vi "controlLaw_deltaU_distEst.vi"(7 "Control Params":T1={"umax"=3.0, "y_ref(k)"=0.0, "Ki"=0.0, "y(k) (from plant)"=0.0, "ND"=0, "NS"=0, "u_Kx_ref(k)"=0.0, "du_max"=3.0, "NS_obs"=0, "NS_control"=0} {"du_max" format="%#_13g"; "u_Kx_ref(k)" format="%#_13g"; "Ki" format="%#_13g"; "y_ref(k)" format="%#_13g"; "umax" format="%#_13g"}, 8 "x^(k)":sgl[](array[numeric])=[0.0, 0.0, 0.0, 0.0, 0.0, 0.0, 0.0, 0.0, 0.0, 0.0, 0.0, 0.0, 0.0, 0.0, 0.0, 0.0, 0.0, 0.0, 0.0, 0.0, 0.0, 0.0, 0.0, 0.0, 0.0]) -> (0 "x^(k+1) = Ax + Bu + Lye":sgl[](array[numeric]), 3 "u(k) (saturated)":sgl)   [LabVIEW 2017]
uses:
  controls/controlParams_tracktraj.ctl
panel:
  out "has_saturated":bool
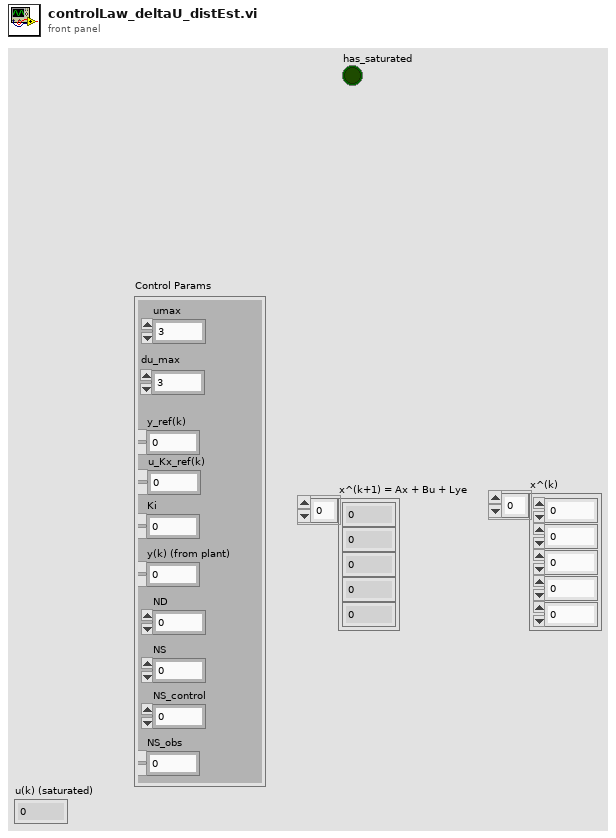
[diagram p1: front panel]
types:
  T1 = typedef "controlParams_tracktraj.ctl" = cluster{"umax":sgl, "y_ref(k)":sgl, "Ki":sgl, "y(k) (from plant)":sgl, "ND":i16, "NS":i16, "u_Kx_ref(k)":sgl, "du_max":sgl, "NS_obs":i16, "NS_control":i16}
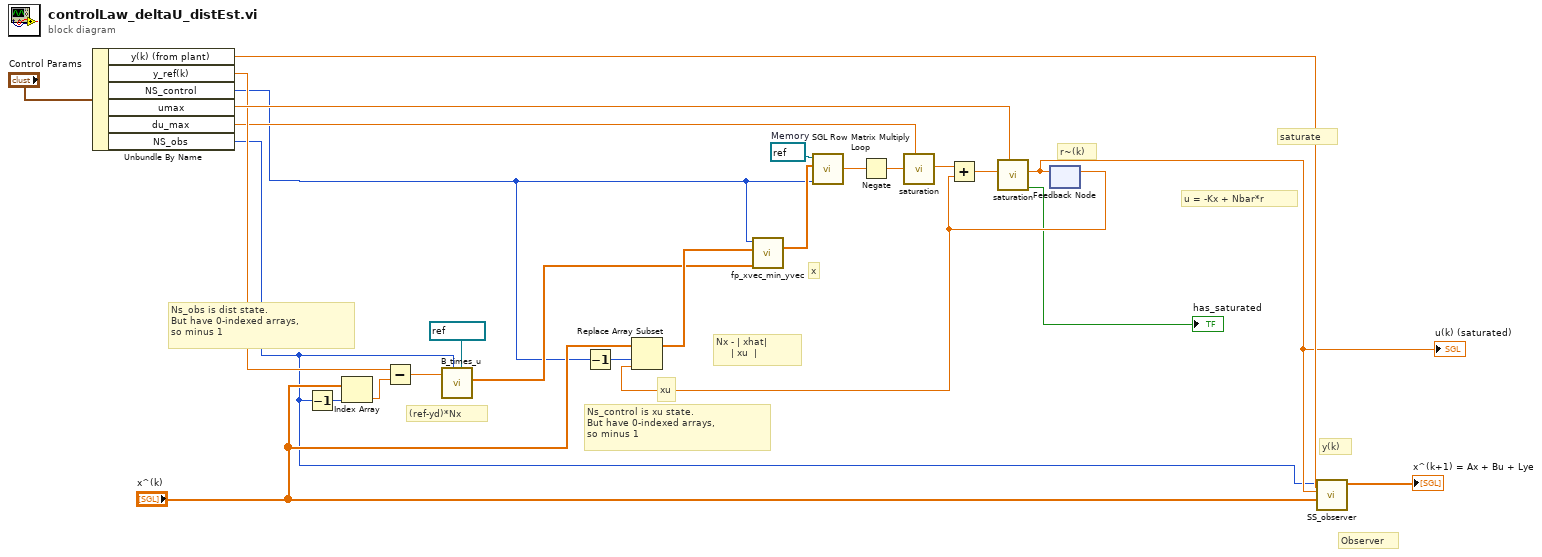
[diagram p0: block diagram]
diagram:
  w25 = refnum<k21> "K"  # Memory
  # "Ns_control is xu state.\nBut have 0-indexed arrays,\nso minus 1"
  # "(ref-yd)*Nx"
  # "xu"
  # "Nx - | xhat|\n     | xu  |"
  # "x"
  # "Ns_obs is dist state.\nBut have 0-indexed arrays,\nso minus 1"
  # "y(k)"
  # "r~(k)"
  # "saturate"
  # "u = -Kx + Nbar*r"
  # "Observer"
  n1 = Unbundle By Name("Control Params") -> ("y(k) (from plant)"=w22:sgl, "y_ref(k)"=w19:sgl, "NS_control"=w1:i16, "umax"=w24:sgl, "du_max"=w7:sgl, "NS_obs"=w2:i16)
  n2 = Decrement(x=w2) -> (x-1=w10:i16)
  n3 = Index Array(array="x^(k)", index=w10) -> (element=w21:sgl)
  n4 = Subtract(x=w19, y=w21) -> (x-y=w20:sgl)
  n5 = call "B_times_u.vi"("Memory"=refnum<k21> "Nx_x", "NS"=w2, "u"=w20) -> ("product(vector)"=w11:sgl[])  [unwired: 8 in]
  n6 = Decrement(x=w1) -> (x-1=w6:i16)
  n7 = feedback #1() -> (w16:sgl)  [unwired: 1 in]
  n8 = Replace Array Subset(array="x^(k)", new element=w16, index=w6) -> (w12:sgl[])
  n9 = call "fp_xvec_min_yvec.vi"("y_vec"=w11, "x_vec"=w12, "N"=w1) -> ("xvec-yvec"=w13:sgl[])  [unwired: 8 in]
  n10 = call "SGL Row Matrix Multiply Loop.vi"("NS"=w1, "X"=w13, "Refnum in"=w25) -> ("Numeric"=w4:sgl)  [unwired: 8 in]
  n11 = Negate(x=w4) -> (-x=w5:sgl)
  n12 = call "saturation.vi"("uMax"=w7, "signal in"=w5) -> ("signal out"=w8:sgl)  [unwired: 8 in, 1 out]
  n13 = Add(x=w8, y=w16) -> (x+y=w17:sgl)
  n14 = call "saturation.vi"("uMax"=w24, "signal in"=w17) -> ("has_saturated"=→"has_saturated":bool, "signal out"=w14:sgl)  [unwired: 8 in]
  "u(k) (saturated)" <- w14
  n15 = feedback-in #1(w14) -> ()
  n16 = call "SS_observer.vi"("y(k)"=w22, "X"="x^(k)", "u(k)"=w14, "NS"=w2) -> ("Ax + Bu + Lye"=→"x^(k+1) = Ax + Bu + Lye":sgl[])  [unwired: 7 in]
